vi "Multiple write.vi"(8 "error in (no error)":errorcluster, 9 "Sections Data":variant[](array[variant]), 10 "Section Names":string[](array[string]), 11 "Configuration File in":refnum<class "Configuration File.lvclass">) -> (0 "error out":errorcluster, 3 "Configuration File out":refnum<class "Configuration File.lvclass">)   [LabVIEW 2019, in "Configuration File.lvlib" / "Configuration File.lvclass"]
doc: "Use this VI to write multiple tags at once. Helps keep the code clean."
uses:
  Configuration File.lvclass
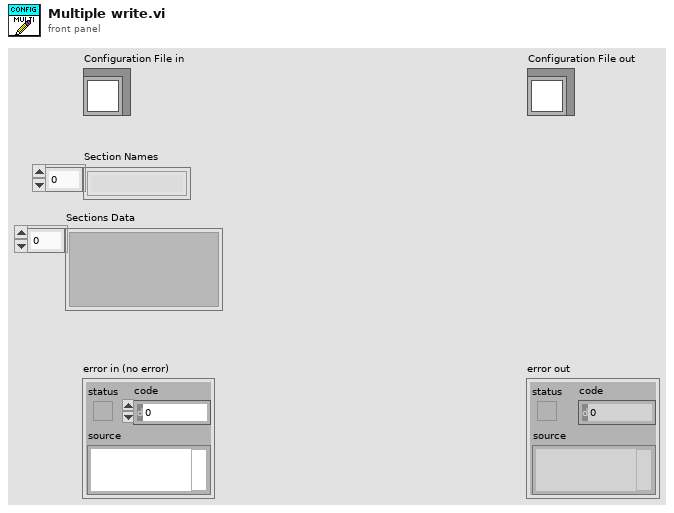
[diagram p1: front panel]
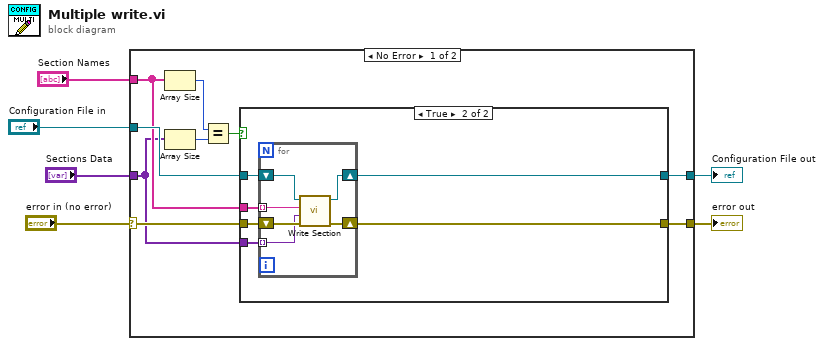
[diagram p0: block diagram]
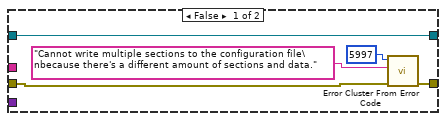
[diagram p2: hidden frame]
diagram:
  n1 = case shown="No Error" "error in (no error)" {
    selector: "error in (no error)" -> [w13 w34]
    tunnel: [w12 w34] -> w5
    tunnel: [w14 w33] -> w3
    tunnel: "Configuration File in" -> [w15 w33]
    tunnel: "Section Names" -> [w11 _]
    tunnel: "Sections Data" -> [w10 _]
    frame No Error {
      n2 = Array Size(array=w11) -> (size(s)=w9:i32)
      n3 = Array Size(array=w10) -> (size(s)=w8:i32)
      n4 = Equal?(x=w9, y=w8) -> (x = y?=w7:bool)
      n5 = case shown="True" w7 {
        tunnel: w15 -> [w20 w26]
        tunnel: [w20 w25] -> w14
        tunnel: w13 -> [w19 w24]
        tunnel: [w18 w23] -> w12
        tunnel: w11 -> [_ w22]
        tunnel: w10 -> [_ w21]
        frame False {
          n6 = call <vilib>:"Error Cluster From Error Code.vi"("error in (no error)"=w19, "error message (\"\")"="Cannot write multiple sections to the configuration file\nbecause there's a different amount of sections and data." ("error message (\"\")"), "error code (0)"=5997) -> ("error out"=w18:errorcluster)  [unwired: 6 in]
        }
        frame True {
          n7 = for {
            tunnel: w22 -> [w28] mode=indexing
            tunnel: w21 -> [w27] mode=indexing
            shift-right: [w31] -> w25
            shift-left: w26 -> [w32]
            shift-right: [w29] -> w23
            shift-left: w24 -> [w30]
            n8 = call-dynamic "Write Section.vi"("error in (no error)"=w30, "Section Data"=w27, "Section Name"=w28, "Configuration File in"=w32) -> ("error out"=w29:errorcluster, "Configuration File out"=w31:refnum<class "Configuration File.lvclass">)  [unwired: 6 in]
          }
        }
      }
    }
    frame Error {
    }
  }
  "error out" <- w5
  "Configuration File out" <- w3
